vi "RGSCoilControl_Wrapper---not_used.vi"() -> ()   [LabVIEW 2018]
panel:
  out "Enable RGS Coils?":bool
  out "Device names":string[](array[string])
  out "Set Values":dbl[](array[numeric])
  in  "Path Array":string[](array[string])
  in  "Input Values":dbl[](array[numeric])
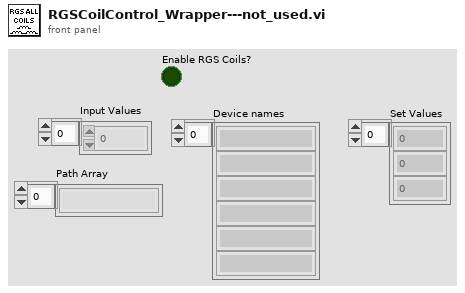
[diagram p1: front panel]
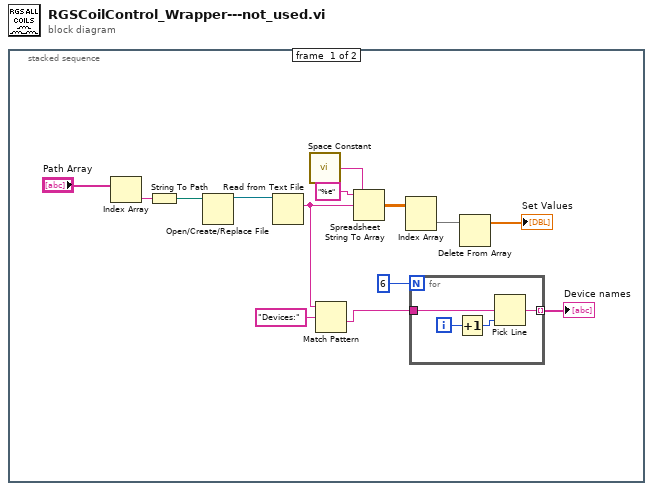
[diagram p0: block diagram]
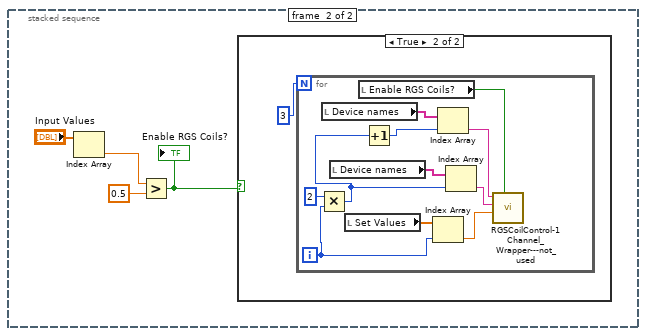
[diagram p2: hidden frame]
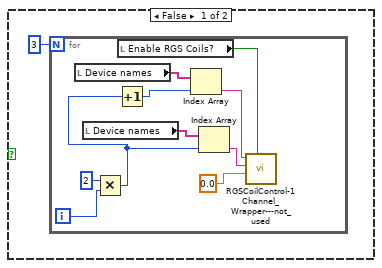
[diagram p3: hidden frame]
diagram:
  n1 = stacked-sequence {
    frame #0 {
      n2 = Index Array(array="Path Array") -> (element=w13:string)  [unwired: 1 in]
      n3 = String To Path(string=w13) -> (path=w1:path)
      n4 = Open/Create/Replace File(file path (use dialog)=w1) -> (refnum out=w3:refnum<file>)  [unwired: 5 in, 2 out]
      n5 = Read from Text File(file (use dialog)=w3) -> (text=w9:string)  [unwired: 3 in, 3 out]
      n6 = call <vilib>:"Space Constant.vi"() -> ("String"=w11:string)
      n7 = Match Pattern(string=w9, regular expression="Devices:") -> (after substring=w7:string)  [unwired: 1 in, 3 out]
      n8 = Spreadsheet String To Array(delimiter (Tab)=w11, format string="%e", spreadsheet string=w9) -> (array=w10:dbl[][])  [unwired: 1 in]
      n9 = Index Array(array=w10) -> (element=w4:dbl[])  [unwired: 2 in]
      n10 = for {
        N: 6 -> [_]
        tunnel: w7 -> [w16]
        tunnel: [w15] -> w5 mode=indexing
        i -> [w18]
        n11 = Increment(x=w18) -> (x+1=w17:i32)
        n12 = Pick Line(multi-line string=w16, line index=w17) -> (output string=w15:string)  [unwired: 1 in]
      }
      "Device names" <- w5
      n13 = Delete From Array(array=w4) -> (array with subset deleted=→"Set Values":dbl[])  [unwired: 2 in, 1 out]
    }
    frame #1 {
      n14 = Index Array(array="Input Values") -> (element=w21:dbl)  [unwired: 1 in]
      n15 = Greater?(x=w21, y=0.5) -> (0:w19:bool)
      "Enable RGS Coils?" <- w19
      n16 = case shown="True" w19 {
        frame False {
          n17 = for {
            N: 3 -> [_]
            i -> [w31]
            n18 = local read "Device names"() -> (w32:string[])
            n19 = local read "Device names"() -> (w33:string[])
            n20 = Multiply(x=2, y=w31) -> (x*y=w28:i32)
            n21 = Increment(x=w28) -> (x+1=w27:i32)
            n22 = local read "Enable RGS Coils?"() -> (w24:bool)
            n23 = Index Array(array=w32, index=w27) -> (element=w26:string)
            n24 = Index Array(array=w33, index=w28) -> (element=w29:string)
            n25 = call "RGSCoilControl-1Channel_Wrapper---not_used.vi"("physical channels"=w26, "lines"=w29, "Current"=0.0, "On/Off"=w24) -> ()  [unwired: 1 in, 1 out]
          }
        }
        frame True {
          n26 = for {
            N: 3 -> [_]
            i -> [w41]
            n27 = Multiply(x=2, y=w41) -> (x*y=w38:i32)
            n28 = local read "Device names"() -> (w43:string[])
            n29 = local read "Device names"() -> (w44:string[])
            n30 = local read "Set Values"() -> (w45:dbl[])
            n31 = local read "Enable RGS Coils?"() -> (w35:bool)
            n32 = Increment(x=w38) -> (x+1=w37:i32)
            n33 = Index Array(array=w45, index=w41) -> (element=w42:dbl)
            n34 = Index Array(array=w43, index=w37) -> (element=w36:string)
            n35 = Index Array(array=w44, index=w38) -> (element=w39:string)
            n36 = call "RGSCoilControl-1Channel_Wrapper---not_used.vi"("physical channels"=w36, "lines"=w39, "Current"=w42, "On/Off"=w35) -> ()  [unwired: 1 in, 1 out]
          }
        }
      }
    }
  }
